vi "DyDisVI.vi"(8 "error in (no error)":errorcluster, 11 "Class1 in":refnum<class "Class1.lvclass">) -> (0 "error out":errorcluster, 3 "Class1 out":refnum<class "Class1.lvclass">)   [LabVIEW 2023, in "Class1.lvclass"]
uses:
  Dynamic Dispatch/Class1.lvclass
  Dynamic Dispatch/Class1.lvclass/Class1.ctl
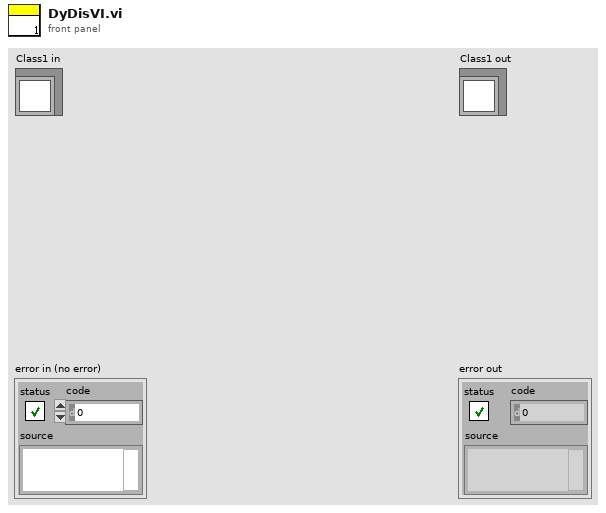
[diagram p1: front panel]
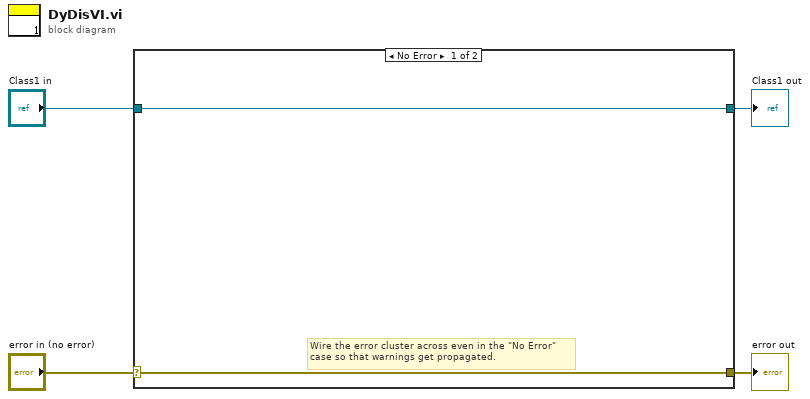
[diagram p0: block diagram]
diagram:
  n1 = case shown="No Error" "error in (no error)" {
    selector: "error in (no error)" -> [w5 w8]
    tunnel: [w5 w8] -> w3
    tunnel: [w6 w7] -> w1
    tunnel: "Class1 in" -> [w6 w7]
    frame No Error {
      # "Wire the error cluster across even in the \"No Error\"\ncase so that warnings get propagated."
    }
    frame Error {
    }
  }
  "error out" <- w3
  "Class1 out" <- w1
